vi "Serialization Test.vi"() -> (0 "validation error":errorcluster, 1 "modules equal":bool, 2 "lines equal before serial test":bool, 3 "lines equal after serial test":bool, 4 "serialization error":errorcluster, 5 "channels equal":bool)   [LabVIEW 2017, in "ActiveFrontEndModule tests.lvlib"]
uses:
  ActiveFrontEndModule tests.lvlib
  module/configuration/ActiveFrontEndModule configuration.lvclass
  C:/Program Files (x86)/National Instruments/LabVIEW 2017/vi.lib/NI/DCAF/Tag Editor Core/control module/configuration/control module configuration.lvclass
  <vilib>/NI/DCAF/Tag Editor Core/control module/configuration/error classification setting.ctl
  <vilib>/NI/Tag Bus Module Framework/runtime/error classification.ctl
  module/configuration/ActiveFrontEndModule configuration.lvclass/ActiveFrontEndModule configuration.ctl
  <vilib>/NI/DCAF/Tag Editor Core/control module/configuration/control module configuration.lvclass/control module configuration.ctl
  <vilib>/NI/DCAF/Tag Editor Core/control module/configuration/Write error classifications.vi
  <vilib>/NI/DCAF/Tag Editor Core/control module/configuration/Read error classifications.vi
  <vilib>/NI/Tag Bus Module Framework/channel/TBM channel.lvclass
  <vilib>/NI/Tag Bus Module Framework/runtime/TBM module execution interface.lvclass
  <vilib>/NI/DCAF/Tag Editor Core/control module/configuration/control module configuration.lvclass
panel:
  out "errors equal after serial test":bool
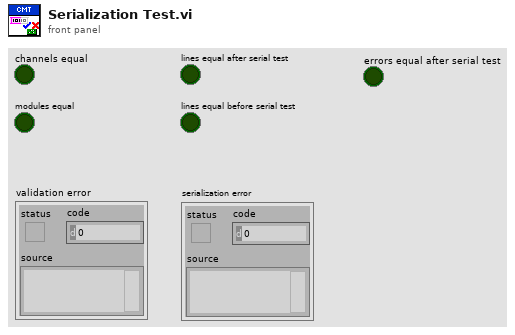
[diagram p1: front panel]
types:
  T1 = typedef "control module configuration.lvclass/error classification setting.ctl" = cluster{"code":i32, "error classification":T2}
  T2 = typedef "TBM module execution interface.lvclass/error classification.ctl" = enum16{"unknown", "none", "trivial", "recoverable", "critical"}
  T3 = cluster{"channel":refnum<class "TBM channel.lvclass">}[]
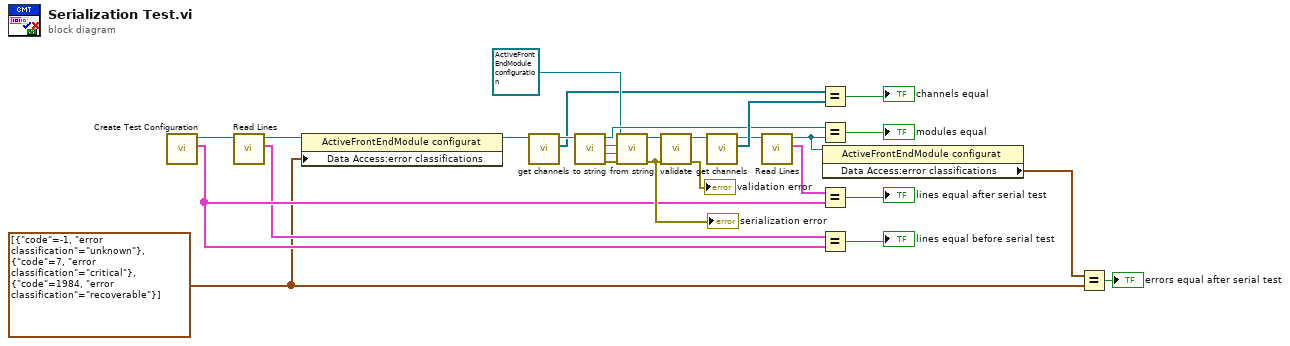
[diagram p0: block diagram]
diagram:
  w4 = T1[] [{"code"=-1, "error classification"=enum."unknown"}, {"code"=7, "error classification"=enum."critical"}, {"code"=1984, "error classification"=enum."recoverable"}] ("error classifications")
  n1 = call "Create Test Configuration.vi"() -> ("Line Array"=w10:T3, "Module"=w27:refnum<class "ActiveFrontEndModule configuration.lvclass">)  [unwired: 6 in, 4 out]
  n2 = call "Read Lines.vi"("ActiveFrontEndModule configuration in"=w27) -> ("Lines"=w9:T3, "ActiveFrontEndModule configuration out"=w5:refnum<class "ActiveFrontEndModule configuration.lvclass">)  [unwired: 8 in, 1 out]
  n3 = property class="ActiveFrontEndModule configurat"(reference=w5, "Data Access:error classifications"=w4) -> (reference out=w1:refnum<class "ActiveFrontEndModule configuration.lvclass">)  [unwired: 1 in, 1 out]
  n4 = call-dynamic "get channels.vi"("fixed channel configuration in"=w1) -> ("channels"=w7:refnum<class "TBM channel.lvclass">[], "fixed channel configuration out"=w13:refnum<class "ActiveFrontEndModule configuration.lvclass">)  [unwired: 9 in]
  n5 = call-dynamic "to string.vi"("fixed channel configuration in"=w13) -> ("error out"=w26:errorcluster, "data"=w25:string, "version"=w24:string, "fixed channel configuration out"=w16:refnum<class "ActiveFrontEndModule configuration.lvclass">)  [unwired: 7 in]
  n6 = call-dynamic "from string.vi"("error in"=w26, "data"=w25, "version"=w24, "fixed channel configuration in"=refnum<class "ActiveFrontEndModule configuration.lvclass"> refnum ("user control module configuration out")) -> ("error out"=w21:errorcluster, "fixed channel configuration out"=w23:refnum<class "ActiveFrontEndModule configuration.lvclass">)  [unwired: 6 in]
  "serialization error" <- w21
  n7 = call-dynamic "validate.vi"("error in"=w21, "fixed channel configuration in"=w23) -> ("error out"=→"validation error":errorcluster, "fixed channel configuration out"=w19:refnum<class "ActiveFrontEndModule configuration.lvclass">)  [unwired: 8 in]
  n8 = call-dynamic "get channels.vi"("fixed channel configuration in"=w19) -> ("channels"=w18:refnum<class "TBM channel.lvclass">[], "fixed channel configuration out"=w11:refnum<class "ActiveFrontEndModule configuration.lvclass">)  [unwired: 9 in]
  n9 = call "Read Lines.vi"("ActiveFrontEndModule configuration in"=w11) -> ("Lines"=w8:T3, "ActiveFrontEndModule configuration out"=w3:refnum<class "ActiveFrontEndModule configuration.lvclass">)  [unwired: 8 in, 1 out]
  n10 = Equal?(x=w7, y=w18) -> (x = y?=→"channels equal":bool)
  n11 = Equal?(x=w16, y=w3) -> (x = y?=→"modules equal":bool)
  n12 = Equal?(x=w8, y=w10) -> (x = y?=→"lines equal after serial test":bool)
  n13 = Equal?(x=w9, y=w10) -> (x = y?=→"lines equal before serial test":bool)
  n14 = property class="ActiveFrontEndModule configurat"(reference=w3) -> ("Data Access:error classifications"=w2:T1[])  [unwired: 1 in, 2 out]
  n15 = Equal?(x=w2, y=w4) -> (x = y?=→"errors equal after serial test":bool)
